vi "Write Justification.vi"(5 "Justification":enum16{"Left", "Center", "Right"}(ring), 9 "Text in":refnum<class "Text.lvclass">) -> (3 "Text out":refnum<class "Text.lvclass">)   [LabVIEW 2014, in "Raspberry Pi Compatible Compiler for LabVIEW.lvlib" / "Text.lvclass"]
uses:
  Text.lvclass
  Text.lvclass/Text.ctl
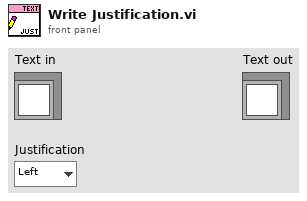
[diagram p1: front panel]
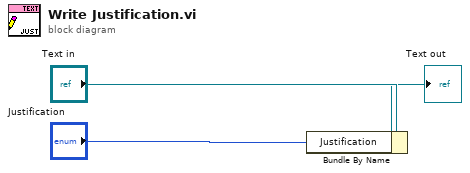
[diagram p0: block diagram]
diagram:
  n1 = Bundle By Name(cluster="Text in", "Justification"="Justification") -> (→"Text out":refnum<class "Text.lvclass">)
